vi "RemoveFromPlaylist.vi"(0 "reference in":refnum<class "MusicPlayer.lvclass">, 7 "File Path":path, 11 "Error In":errorcluster) -> (4 "reference out":refnum<class "MusicPlayer.lvclass">, 15 "Error Out":errorcluster)   [LabVIEW 2022 SP3, in "MusicPlayer.lvclass"]
uses:
  MusicPlayer.lvclass
  MusicPlayer.lvclass/MusicPlayer.ctl
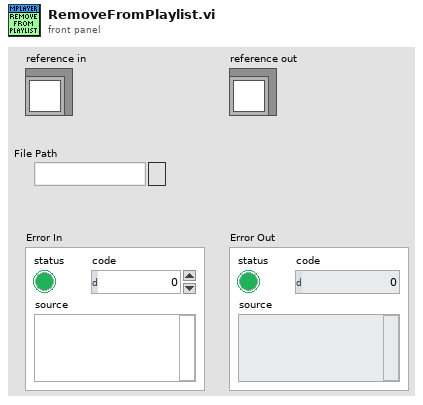
[diagram p1: front panel]
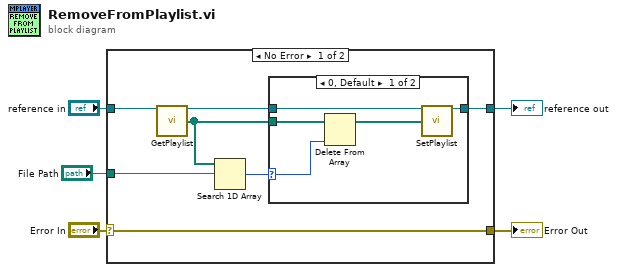
[diagram p0: block diagram]
diagram:
  n1 = case shown="No Error" "Error In" {
    selector: "Error In" -> [w12 w20]
    tunnel: [w12 w20] -> w4
    tunnel: [w10 w19] -> w2
    tunnel: "reference in" -> [w11 w19]
    tunnel: "File Path" -> [w8 _]
    frame No Error {
      n2 = call "GetPlaylist.vi"("reference in"=w11) -> ("reference out"=w9:refnum<class "MusicPlayer.lvclass">, "Playlist"=w6:path[])  [unwired: 12 in, 1 out]
      n3 = Search 1D Array(1D array=w6, element=w8) -> (index of element=w7:i32)  [unwired: 1 in]
      n4 = case shown="0, Default" w7 {
        selector: w7 -> [w14 _]
        tunnel: [w17 w18] -> w10
        tunnel: w9 -> [w16 w18]
        tunnel: w6 -> [w15 _]
        frame 0, Default {
          n5 = Delete From Array(array=w15, index=w14) -> (array with subset deleted=w13:path[])  [unwired: 1 in, 1 out]
          n6 = call "SetPlaylist.vi"("reference in"=w16, "Playlist"=w13) -> ("reference out"=w17:refnum<class "MusicPlayer.lvclass">)  [unwired: 12 in, 1 out]
        }
        frame -1 {
        }
      }
    }
    frame Error {
    }
  }
  "Error Out" <- w4
  "reference out" <- w2
